vi "Read Port.vi"(8 "error in (no error)":errorcluster, 11 "Handle":u32) -> (0 "error out":errorcluster, 2 "function return":i32, 3 "Data":u8)   [LabVIEW 2014, in "Photon Counter.lvlib" / "C8855-01.lvlib"]
doc: "BOOL C8855API __stdcall C8855ReadPort( HANDLE hC8855,\n BYTE *Data );"
uses:
  C8855-01.lvlib
  C8855-01api.dll
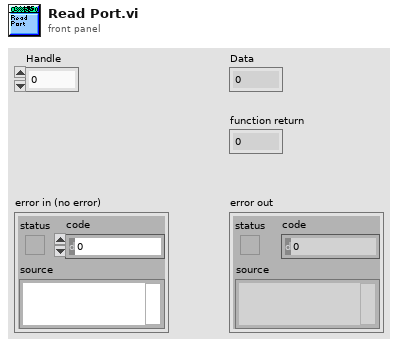
[diagram p1: front panel]
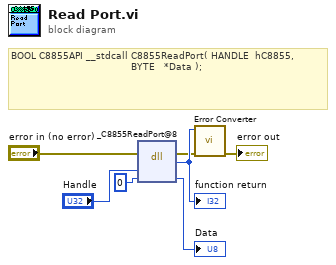
[diagram p0: block diagram]
diagram:
  # "BOOL C8855API __stdcall C8855ReadPort( HANDLE  hC8855,\n                                        BYTE   *Data );"
  n1 = dll-call lib="C:/Users/Andy/Desktop/Trace Grabber/Drivers/C8855-01/C8855-01api.*" fn="_C8855ReadPort@8"(error in="error in (no error)", "Handle"="Handle", "Data"=u8 0) -> (error out=w2:errorcluster, w7:i32, "Data"=→"Data":u8)  [unwired: 3 in, 1 out]
  "function return" <- w7
  n2 = call "Error Converter.vi"("error in (no error)"=w2, "error code"=w7) -> ("error out"=→"error out":errorcluster)  [unwired: 9 in]
